vi "Template_MouseDown.vi"(7 "Add to Undo?":bool=TRUE, 8 "error in":errorcluster, 10 "CtlRef":refnum<vi>, 11 "Data in":T1={"Class"={"Ants"=refnum, "Layer"=refnum, "Templates"=refnum, "Icon"=refnum, "Glyph"=refnum, "Settings"=refnum, "Tools"=refnum, "History"=refnum}, "Ref"={"Add Layer"=refnum, "Remove Layer"=refnum, "Line Text"=[], "Body Text Spec"=refnum, "DNL_Font"=refnum, "glyph path str"=refnum, "templates path str"=refnum, "Arrow Up"=refnum, "Arrow Down"=refnum, "IE VI Ref"=refnum, "Glyphs tree"=refnum, "Templates tree"=refnum, "Layer Icon Text"=refnum, "Layer Template"=refnum, "Body Text"=refnum, "Search Templates"=refnum, "TextMarker"=refnum, "Tab Control"=refnum, "Search Glyphs"=refnum, "Line Color"=refnum, "DNL_Glyphs []"=refnum, "Fill Color"=refnum, "Tools"=refnum, "Icon"=refnum, "Preview"=refnum, "Ants"=refnum, "Terminals"=refnum, "menu reference"=refnum, "LayerNames"=[], "GlyphLoadAnimation"=refnum, "TemplateLoadAnimation"=refnum, "refreshGlyphs"=refnum, "refreshTemplates"=refnum}, "Support"={"AntsRect"={"left"=0, "top"=0, "right"=0, "bottom"=0}, "Mouse Move Coords"={"Horizontal"=0, "Vertical"=0}, "Mouse Down Coords"={"Horizontal"=0, "Vertical"=0}, "Temp Coord"={"Horizontal"=0, "Vertical"=0}, "Action"=enum."Default", "Edge Color"=4914962, "Fill Color"=16860, "Mouse Down?"=FALSE, "Draft Mode?"=FALSE, "Temp Icon"=bytes[3102], "CTRL Pressed"=FALSE, "Move Selection?"=FALSE, "AntsRect Orig"={"left"=0, "top"=0, "right"=0, "bottom"=0}, "Text"="", "TM Set?"=FALSE, "Mouse inside icon?"=FALSE, "Tool (old value)"=0, "Pencil Move Color"=0, "Swap Colors?"=FALSE, "Shift pressed?"=FALSE}}) -> (0 "error out":errorcluster, 3 "Data out":T1={"Class"={"Ants"=refnum, "Layer"=refnum, "Templates"=refnum, "Icon"=refnum, "Glyph"=refnum, "Settings"=refnum, "Tools"=refnum, "History"=refnum}, "Ref"={"Add Layer"=refnum, "Remove Layer"=refnum, "Line Text"=[], "Body Text Spec"=refnum, "DNL_Font"=refnum, "glyph path str"=refnum, "templates path str"=refnum, "Arrow Up"=refnum, "Arrow Down"=refnum, "IE VI Ref"=refnum, "Glyphs tree"=refnum, "Templates tree"=refnum, "Layer Icon Text"=refnum, "Layer Template"=refnum, "Body Text"=refnum, "Search Templates"=refnum, "TextMarker"=refnum, "Tab Control"=refnum, "Search Glyphs"=refnum, "Line Color"=refnum, "DNL_Glyphs []"=refnum, "Fill Color"=refnum, "Tools"=refnum, "Icon"=refnum, "Preview"=refnum, "Ants"=refnum, "Terminals"=refnum, "menu reference"=refnum, "LayerNames"=[], "GlyphLoadAnimation"=refnum, "TemplateLoadAnimation"=refnum, "refreshGlyphs"=refnum, "refreshTemplates"=refnum}, "Support"={"AntsRect"={"left"=0, "top"=0, "right"=0, "bottom"=0}, "Mouse Move Coords"={"Horizontal"=0, "Vertical"=0}, "Mouse Down Coords"={"Horizontal"=0, "Vertical"=0}, "Temp Coord"={"Horizontal"=0, "Vertical"=0}, "Action"=enum."Default", "Edge Color"=4914962, "Fill Color"=16860, "Mouse Down?"=FALSE, "Draft Mode?"=FALSE, "Temp Icon"=bytes[3102], "CTRL Pressed"=FALSE, "Move Selection?"=FALSE, "AntsRect Orig"={"left"=0, "top"=0, "right"=0, "bottom"=0}, "Text"="", "TM Set?"=FALSE, "Mouse inside icon?"=FALSE, "Tool (old value)"=0, "Pencil Move Color"=0, "Swap Colors?"=FALSE, "Shift pressed?"=FALSE}})   [LabVIEW 2020]
uses:
  Class/Ants/Ants.lvclass
  Class/FakedArray/FakedArray.lvclass
  vi.lib/LabVIEW Icon API/lv_icon/Classes/Icon/Icon.lvclass
  Class/Icon Library/Glyph.lvclass
  Class/Settings/Settings.lvclass
  Class/Tools/Tools Paint.lvclass
  vi.lib/LabVIEW Icon API/lv_icon/Classes/Icon Framework/Icon Framework.lvclass
  vi.lib/LabVIEW Icon API/lv_icon/Controls/LayerType.ctl
  History/History.lvlib
  <vilib>/Utility/miscctls.llb/LVPoint32TypeDef.ctl
  Controls/SupportClass_Action.ctl
  vi.lib/LabVIEW Icon API/lv_icon/Controls/IEColor.ctl
  Controls/Support Cluster.ctl
  lv_icon.lvlib
  Controls/References Cluster.ctl
  Controls/IE Classes.ctl
  Controls/Global Data.ctl
  History/History/History.lvclass
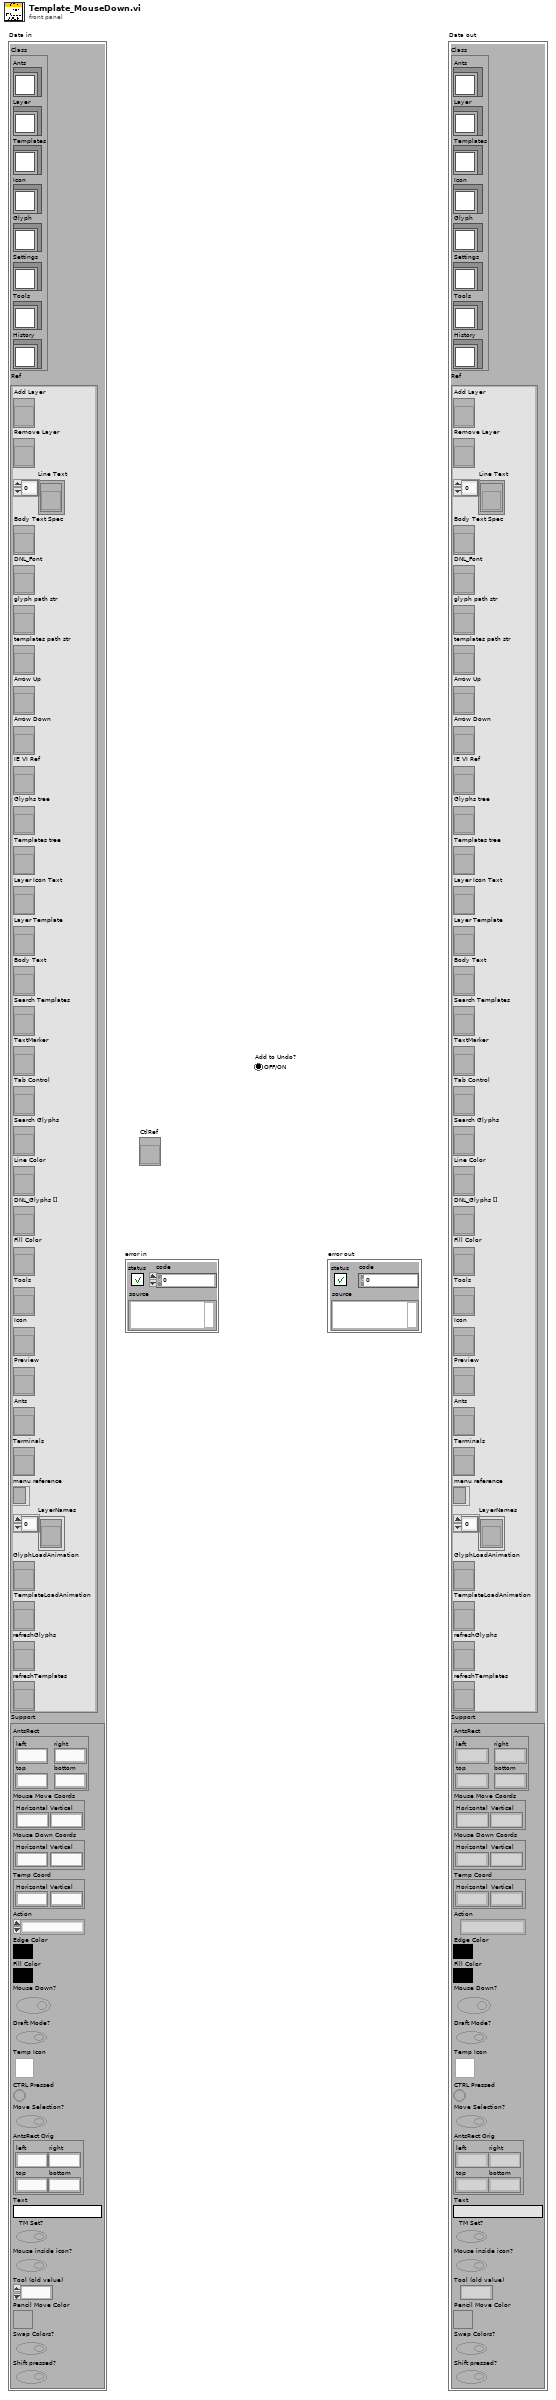
[diagram p1: front panel]
types:
  T1 = typedef "lv_icon.lvlib/Global Data.ctl" = cluster{"Class":T2, "Ref":T3, "Support":T4}
  T2 = typedef "lv_icon.lvlib/IE Classes.ctl" = cluster{"Ants":refnum<class "Ants.lvclass">, "Layer":refnum<class "FakedArray.lvclass">, "Templates":refnum<class "FakedArray.lvclass">, "Icon":refnum<class "Icon.lvclass">, "Glyph":refnum<class "Glyph.lvclass">, "Settings":refnum<class "Settings.lvclass">, "Tools":refnum<class "Tools Paint.lvclass">, "History":refnum<class "History.lvclass">}
  T3 = typedef "lv_icon.lvlib/References Cluster.ctl" = cluster{"Add Layer":refnum<vi>, "Remove Layer":refnum<vi>, "Line Text":refnum<vi>[], "Body Text Spec":refnum<vi>, "DNL_Font":refnum<vi>, "glyph path str":refnum<vi>, "templates path str":refnum<vi>, "Arrow Up":refnum<vi>, "Arrow Down":refnum<vi>, "IE VI Ref":refnum<vi>, "Glyphs tree":refnum<vi>, "Templates tree":refnum<vi>, "Layer Icon Text":refnum<vi>, "Layer Template":refnum<vi>, "Body Text":refnum<vi>, "Search Templates":refnum<vi>, "TextMarker":refnum<vi>, "Tab Control":refnum<vi>, "Search Glyphs":refnum<vi>, "Line Color":refnum<vi>, "DNL_Glyphs []":refnum<vi>, "Fill Color":refnum<vi>, "Tools":refnum<vi>, "Icon":refnum<vi>, "Preview":refnum<vi>, "Ants":refnum<vi>, "Terminals":refnum<vi>, "menu reference":refnum<k9>, "LayerNames":refnum<vi>[], "GlyphLoadAnimation":refnum<vi>, "TemplateLoadAnimation":refnum<vi>, "refreshGlyphs":refnum<vi>, "refreshTemplates":refnum<vi>}
  T4 = typedef "lv_icon.lvlib/Support Cluster.ctl" = cluster{"AntsRect":cluster{"left":i16, "top":i16, "right":i16, "bottom":i16}, "Mouse Move Coords":T5, "Mouse Down Coords":T5, "Temp Coord":T5, "Action":T6, "Edge Color":T7, "Fill Color":T7, "Mouse Down?":bool, "Draft Mode?":bool, "Temp Icon":picture, "CTRL Pressed":bool, "Move Selection?":bool, "AntsRect Orig":cluster{"left":i16, "top":i16, "right":i16, "bottom":i16}, "Text":string, "TM Set?":bool, "Mouse inside icon?":bool, "Tool (old value)":u32, "Pencil Move Color":u32, "Swap Colors?":bool, "Shift pressed?":bool}
  T5 = typedef "LVPoint32TypeDef.ctl" = cluster{"Horizontal":i32, "Vertical":i32}
  T6 = typedef "SupportClass_Action.ctl" = enum16{"Default", "Move Selection", "Glyph Library", "Tool"}
  T7 = typedef "IEColor.ctl" = u32
  T8 = typedef "LayerType.ctl" = enum16{"Graphic", "Text", "Tool", "Graphic Drop"}
  T9 = typedef "Graphic.ctl" = cluster{"Rectangle":cluster{"left":i16, "top":i16, "right":i16, "bottom":i16}, "Path":path, "Image":picture, "Filter":string, "FileName":string}
  T10 = typedef "Layer.ctl" = cluster{"LayerIcon":picture, "LayerName":string, "Opacity":u8, "Visibility?":bool}
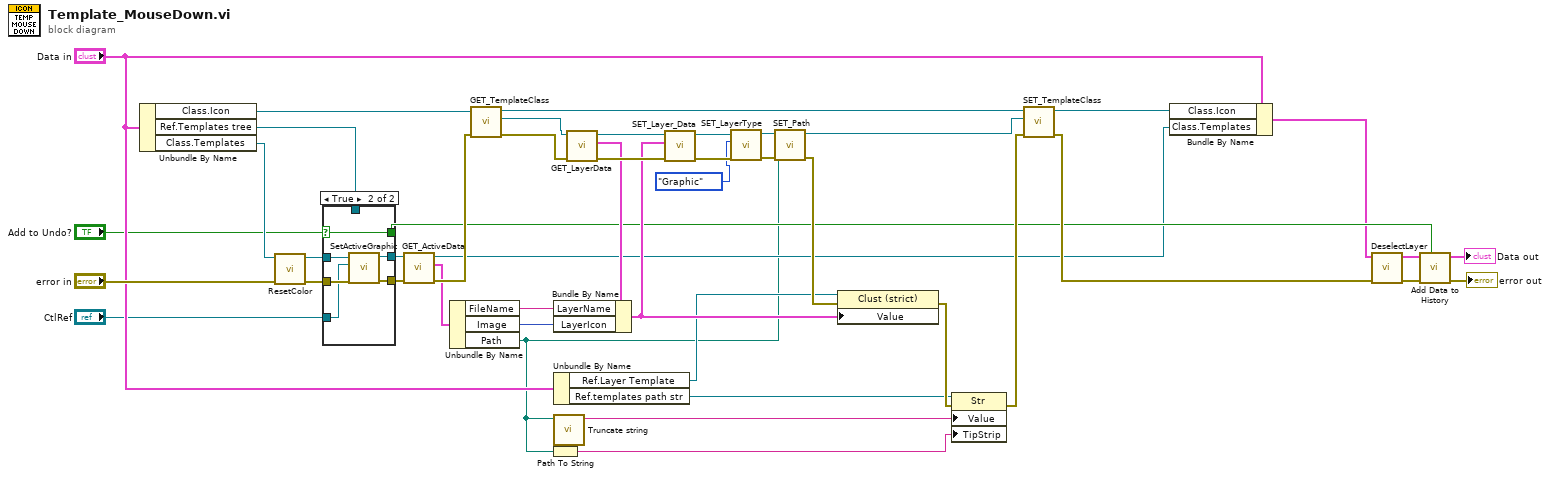
[diagram p0: block diagram]
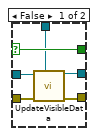
[diagram p2: hidden frame]
diagram:
  n1 = Unbundle By Name("Data in") -> ("Class.Icon"=w14:refnum<class "Icon.lvclass">, "Ref.Templates tree"=w6:refnum<vi>, "Class.Templates"=w12:refnum<class "FakedArray.lvclass">)
  n2 = call "ResetColor.vi"("error in (no error)"="error in", "FakedArray in"=w12) -> ("error out"=w41:errorcluster, "FakedArray out"=w22:refnum<class "FakedArray.lvclass">)  [unwired: 8 out]
  n3 = case shown="True" "Add to Undo?" {
    selector: "Add to Undo?" -> [w49 w52]
    tunnel: "CtlRef" -> [_ w55]
    tunnel: [w48 w54] -> w31
    tunnel: [w50 w57] -> w45
    tunnel: w22 -> [w47 w53]
    tunnel: w41 -> [w51 w56]
    tunnel: [w49 w52] -> w19
    tunnel: w6 -> [w46 _]
    frame False {
      n4 = call-dynamic "UpdateVisibleData.vi"("Templates tree"=w46, "error in (no error)"=w51, "FakedArray in"=w47) -> ("error out"=w50:errorcluster, "FakedArray out"=w48:refnum<class "FakedArray.lvclass">)  [unwired: 2 in, 5 out]
    }
    frame True {
      n5 = call-dynamic "SetActiveGraphic.vi"("error in (no error)"=w56, "Ctl Refnum"=w55, "FakedArray in"=w53) -> ("error out"=w57:errorcluster, "FakedArray out"=w54:refnum<class "FakedArray.lvclass">)  [unwired: 3 in, 4 out]
    }
  }
  n6 = call-dynamic "GET_ActiveData.vi"("error in (no error)"=w45, "FakedArray in"=w31) -> ("error out"=w42:errorcluster, "Path & Icon"=w20:T9, "FakedArray out"=w11:refnum<class "FakedArray.lvclass">)  [unwired: 7 out]
  n7 = Unbundle By Name(w20) -> ("FileName"=w16:string, "Image"=w30:picture, "Path"=w3:path)
  n8 = call-dynamic "GET_TemplateClass.vi"("error in (no error)"=w42, "Icon.lvclass in"=w14) -> ("error out"=w40:errorcluster, "Icon Framework.lvclass"=w23:refnum<class "Icon Framework.lvclass">, "Icon.lvclass out"=w25:refnum<class "Icon.lvclass">)  [unwired: 7 out]
  n9 = Path To String(path=w3) -> (string=w15:string)
  n10 = Unbundle By Name("Data in") -> ("Ref.Layer Template"=w21:refnum<vi>, "Ref.templates path str"=w18:refnum<vi>)
  n11 = call "Truncate string.vi"("File Path"=w3) -> ("String path out"=w17:string)  [unwired: 1 in, 9 out]
  n12 = call-dynamic "GET_LayerData.vi"("error in (no error)"=w40, "Layer.lvclass in"=w23) -> ("error out"=w43:errorcluster, "Data"=w26:T10, "Layer.lvclass out"=w27:refnum<class "Icon Framework.lvclass">)  [unwired: 7 out]
  n13 = Bundle By Name(cluster=w26, "LayerName"=w16, "LayerIcon"=w30) -> (w24:T10)
  n14 = call-dynamic "SET_Layer_Data.vi"("error in (no error)"=w43, "Data"=w24, "Layer.lvclass in"=w27) -> ("error out"=w44:errorcluster, "Layer.lvclass out"=w28:refnum<class "Icon Framework.lvclass">)  [unwired: 1 in, 6 out]
  n15 = call-dynamic "SET_LayerType.vi"("error in (no error)"=w44, "Type"=LayerType."Graphic", "Layer.lvclass in"=w28) -> ("error out"=w33:errorcluster, "Layer.lvclass out"=w5:refnum<class "Icon Framework.lvclass">)  [unwired: 7 out]
  n16 = call "SET_Path.vi"("error in (no error)"=w33, "Path"=w3, "Icon Framework.lvclass in"=w5) -> ("error out"=w32:errorcluster, "Icon Framework.lvclass out"=w4:refnum<class "Icon Framework.lvclass">)  [unwired: 7 in]
  n17 = property class="Clust (strict)"(reference=w21, error in=w32, "Value"=w24) -> (error out=w37:errorcluster)  [unwired: 1 out]
  n18 = property class="Str"(reference=w18, error in=w37, "Value"=w17, "TipStrip"=w15) -> (error out=w36:errorcluster)  [unwired: 1 out]
  n19 = call-dynamic "SET_TemplateClass.vi"("error in (no error)"=w36, "Icon Framework.lvclass"=w4, "Icon.lvclass in"=w25) -> ("error out"=w35:errorcluster, "Icon.lvclass out"=w13:refnum<class "Icon.lvclass">)  [unwired: 7 out]
  n20 = Bundle By Name(cluster="Data in", "Class.Icon"=w13, "Class.Templates"=w11) -> (w10:T1)
  n21 = call "DeselectLayer.vi"("error in (no error)"=w35, "Data in"=w10) -> ("error out"=w39:errorcluster, "Data out"=w9:T1)  [unwired: 8 out]
  n22 = call "Add Data to History.vi"(7:w19, "error in"=w39, "Data in"=w9) -> ("error out"=→"error out":errorcluster, "Data out"=→"Data out":T1)  [unwired: 7 out]
